vi "Run Bitfile.vi"() -> ()   [LabVIEW 2011]
uses:
  <vilib>/Platform/TimedLoop/XDataNode/timing_clust.ctl
  <vilib>/Platform/TimedLoop/XDataNode/nitl_modes.ctl
  <vilib>/Platform/TimedLoop/XDataNode/wakeup.ctl
  <vilib>/FPGAPlugInAG/sbRIO-9606/niLvFpga_Open_sbRIO-9606.vi
  <vilib>/rvi/interface/common/dynamic/niFpgaDynamicAddResources.vi
  <vilib>/Utility/error.llb/Error Cluster From Error Code.vi
  <vilib>/rvi/errors/niLvFpgaAdjustHostInterfaceError.vi
  <vilib>/FPGAPlugInAG/Dynamic/niLvFpga_Close_Dynamic.vi
  <vilib>/Platform/TimedLoop/XDataNode/XDataNode.xnode
  <vilib>/rvi/interface/nirviOpenFPGA/nirviOpenFPGA.xnode
  FPGA Bitfiles/natcar_FPGATarget_Top-Level_610FB000.lvbitx
  <vilib>/rvi/interface/nirviReadWriteControl/nirviReadWriteControl.xnode
  <vilib>/rvi/interface/nirviCloseFPGA/nirviCloseFPGA.xnode
  <vilib>/Platform/TimedLoop/XDataNode/XDNodeRunTimeDep.lvlib
  NiFpgaLv.dll
  <vilib>/rvi/interface/Simulation/niFpgaSimulationCallBeginRW.vi
panel:
  out "straight":bool
  in  "slow":u16=45 max=100 step=1
  in  "fast":u16=53 max=100 step=1
  out "using SL,SR":bool
  out "Error from SL,SR":dbl(graph)
  out "from SL,SR":dbl
  out "S5":bool
  out "S4":bool
  out "S2":bool
  out "S1":bool
  out "Raw Sensor Data":T1(graph)
  out "Go Duty":u16
  out "Servo 1e-7s":u32
  out "Line Error Graph":dbl(graph)
  out "Error (cm)":dbl
  in  "Steering Kp":dbl=270.0 min=0.0 max=1000.0 step=1.0
  out "really lost":bool
  out "line found":bool
  out "SC":bool
  out "S3":bool
  out "AI7":u16
  out "AI6":u16
  out "AI5":u16
  out "AI4":u16
  out "AI3":u16
  out "AI2":u16
  out "AI1":u16
  out "AI0":u16
  out "Speed Error":dbl(graph)
  in  "Offset":dbl=35.0 min=0.0 max=30.0 step=0.1
  out "Velocity counts":u32
  out "V [m/s]":dbl
  in  "RUN!":bool
  in  "Stop":bool
  in  "Kff":dbl=6.0 min=0.0 max=10.0 step=0.1
  in  "uBlaze Reset":bool
  in  "Steering ON 1e-7s":u32=15000 min=10240 max=19650 step=100
  in  "Steering":bool
  in  "Throttle":bool
  in  "GO frequency (Hz)":u16=1000 min=10 max=10000 step=10
  in  "GO duty":u16 max=100 step=1
  in  "Vdes [m/s]":dbl min=0.0 max=5.0 step=0.1
  in  "Speed Ki":dbl=0.1 min=0.0 max=2.0 step=0.01
  in  "Throttle ON":bool
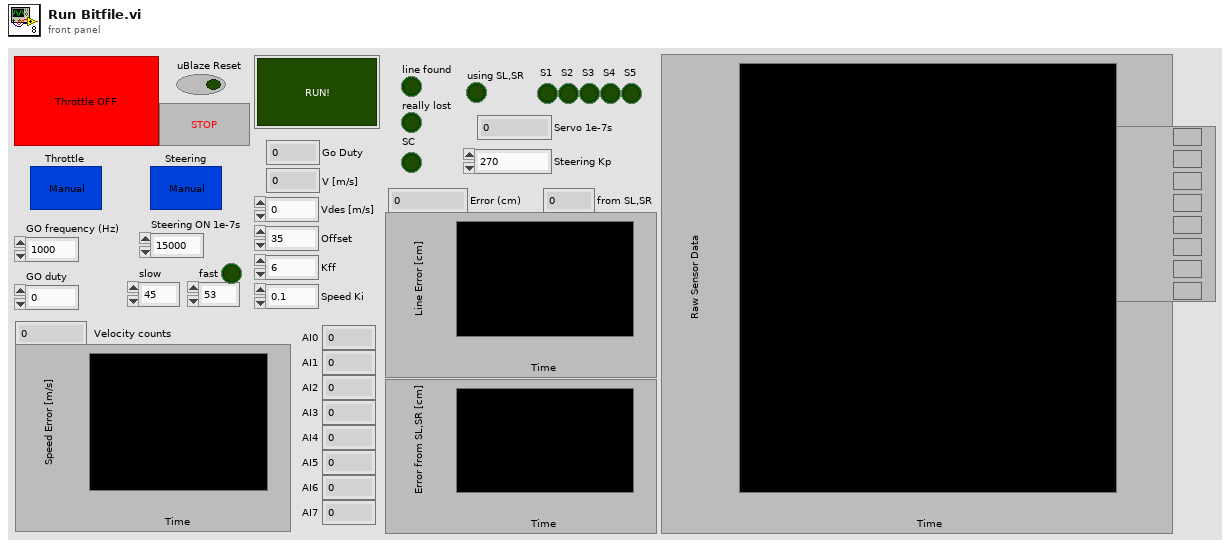
[diagram p1: front panel]
types:
  T1 = cluster{"AI0":u16, "AI1":u16, "AI2":u16, "AI3":u16, "AI4":u16, "AI5":u16, "AI6":u16, "AI7":u16}
  T2 = typedef "XDNodeRunTimeDep.lvlib/timing_clust.ctl" = cluster{"Expected End [f-1]":u64, "Actual End [f-1]":u64, "Finished Late? [f-1]":bool, "Expected End [i-1]":u64, "Actual End [i-1]":u64, "Finished Late? [i-1]":bool, "Expected Start [i]":u64, "Actual Start [i]":u64, "Expected Start [f]":u64, "Actual Start [f]":u64, "Source Name":string, "Structure Name":string, "Period":i64, "Deadline":i64, "Offset":i64, "Start":i64, "Priority":i32, "Timeout":i32, "Mode":T3, "Wakeup Reason":T4, "Error":errorcluster, "Source Type":string, "Secondary Source Type":string, "Global End Time":u64, "Global Start Time":u64, "Frame Duration":u64, "Iteration Duration":u64, "Assigned CPU":i32, "I/O Scan Engine Mode":u32}
  T3 = typedef "XDNodeRunTimeDep.lvlib/nitl_modes.ctl" = enum32{"No Change", "Process missed periods, maintain original phase", "Discard missed periods, maintain original phase", "Process missed periods, ignore original phase", "Discard missed periods, ignore original phase"}
  T4 = typedef "XDNodeRunTimeDep.lvlib/wakeup.ctl" = enum32{"Normal", "Aborted", "Asynchronous wakeup", "Timing source error", "Timed loop error", "Timeout"}
  T5 = cluster{"AI5":u16, "AI6":u16, "AI7":u16, "AI2":u16, "AI1":u16, "AI3":u16, "AI4":u16, "AI0":u16}
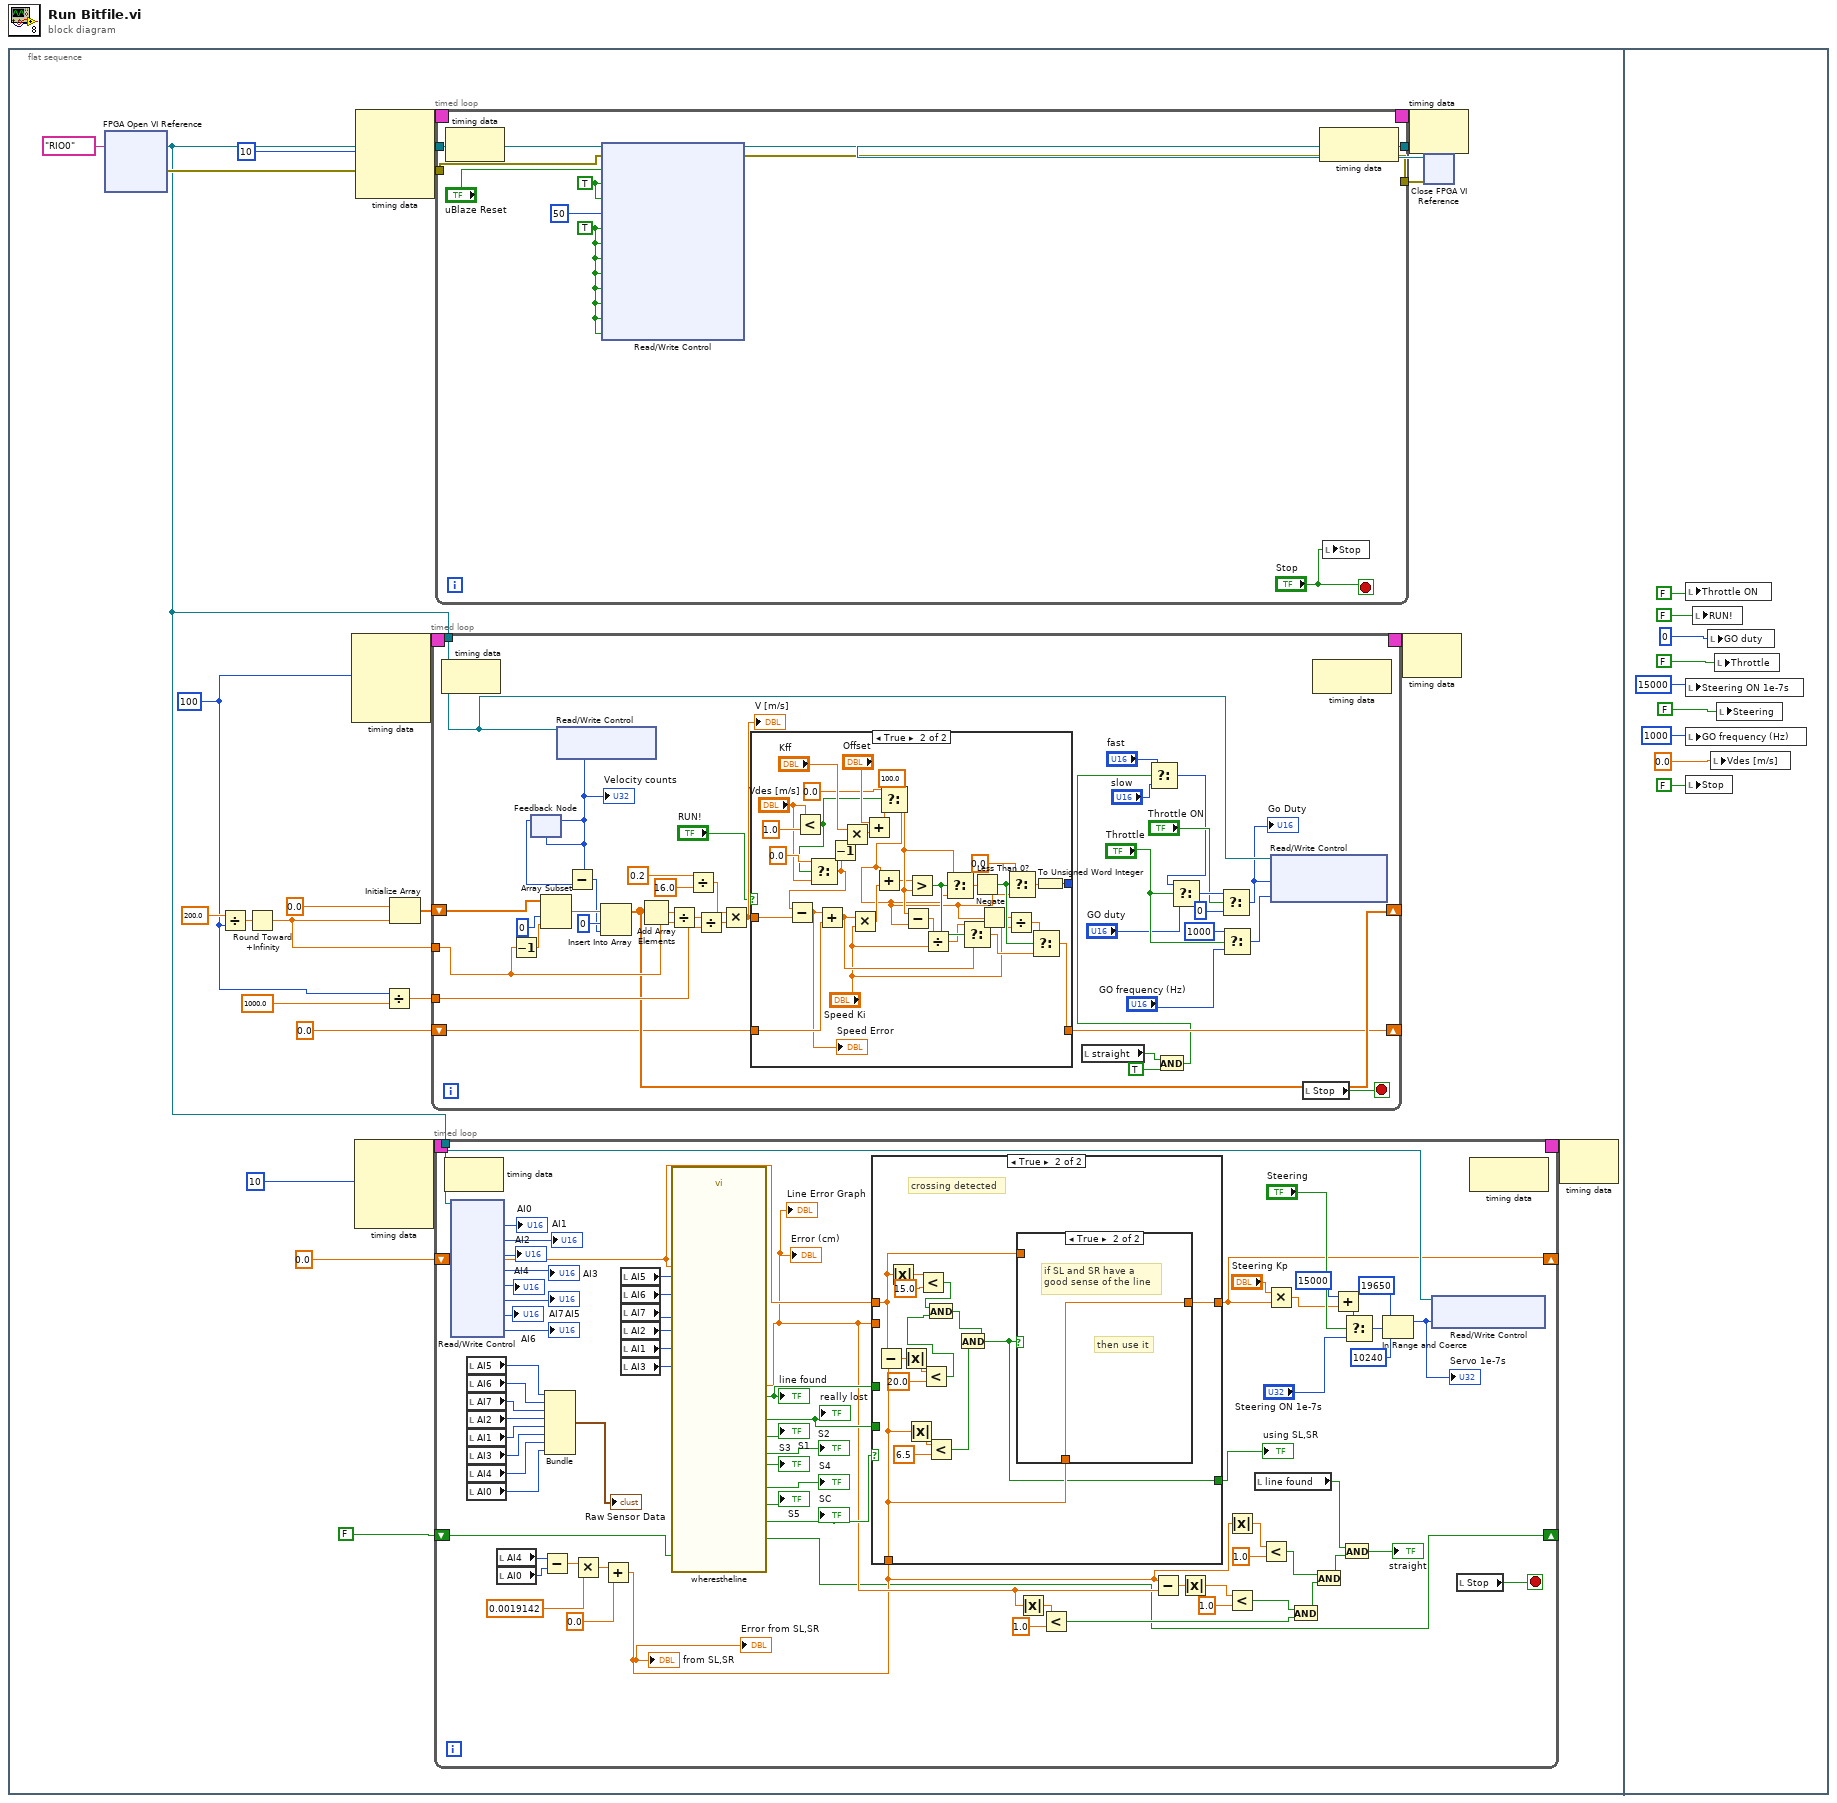
[diagram p0: block diagram]
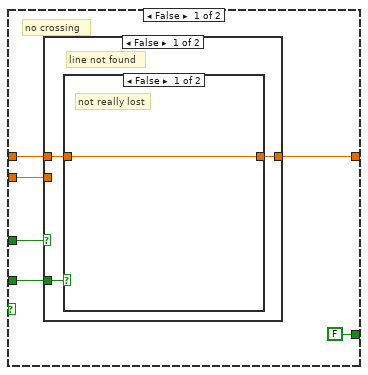
[diagram p2: hidden frame]
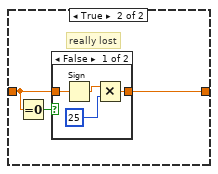
[diagram p3: hidden frame]
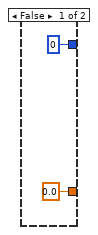
[diagram p7: hidden frame]
diagram:
  n1 = flat-sequence {
    frame #0 {
      w4 = i64 100 ("Period")
      n2 = xnode "FPGA Open VI Reference"("resource name"=tag "RIO0") -> ("FPGA VI Reference Out"=w3:refnum<k20>, "error out"=w17:errorcluster)  [unwired: 1 in]
      n3 = Divide(x=200.0, y=w4) -> (x/y=w11:dbl)
      n4 = Round Toward +Infinity(x=w11) -> (ceil(x): smallest int >= x=w10:dbl)
      n5 = node-c288(w4) -> (w24:T2)  [unwired: 3 in]
      n6 = node-c288(i64 10 ("Period")) -> (w22:T2)  [unwired: 3 in]
      n7 = node-c288(i64 10 ("Period")) -> (w20:T2)  [unwired: 3 in]
      n8 = Divide(x=w4, y=1000.0) -> (x/y=w6:dbl)
      n9 = Initialize Array(0.0 ("element"), w10) -> (w14:dbl[])
      n10 = timed-loop {
        timing: w24 -> [_]
        timing-out: [_] -> w23
        shift-right: [w187] -> _
        shift-left: w14 -> [w186]
        tunnel: w10 -> [w189]
        tunnel: w6 -> [w188]
        shift-right: [w184] -> _
        shift-left: 0.0 -> [w185]
        tunnel: w3 -> [w183]
        stop <- w182 stop-if-true
        n11 = node-c288() -> ()  [unwired: 1 in, 1 out]
        n12 = Decrement(x=w189) -> (x-1=w171:dbl)
        n13 = Array Subset(array=w186, index=0, length=w171) -> (w163:dbl[])
        n14 = xnode "Read/Write Control"("FPGA VI Reference In"=w183) -> ("Velocity counts"=w159:u32)  [unwired: 1 in, 2 out]
        "Velocity counts" <- w159
        n15 = feedback #1(w159) -> (w160:u32)
        n16 = feedback-in #1(w159) -> ()
        n17 = Subtract(x=w159, y=w160) -> (x-y=w162:u32)
        n18 = Insert Into Array(array=w163, index=0, new element=w162) -> (w187:dbl[])
        n19 = Add Array Elements(numeric array=w187) -> (sum=w161:dbl)
        n20 = Divide(x=w161, y=w189) -> (x/y=w169:dbl)
        n21 = Divide(x=0.2, y=16.0) -> (x/y=w165:dbl)
        n22 = Divide(x=w169, y=w188) -> (x/y=w166:dbl)
        n23 = Multiply(x=w165, y=w166) -> (x*y=w164:dbl)
        "V [m/s]" <- w164
        n24 = case shown="True" "RUN!" {
          tunnel: w185 -> [_ w223]
          tunnel: [0.0 w222] -> w184
          tunnel: [u16 0 w221] -> _
          tunnel: w164 -> [_ w220]
          frame False {
          }
          frame True {
            w214 = 100.0 ("y")
            n25 = Less?(x="Vdes [m/s]", y=1.0) -> (x < y?=w196:bool)
            n26 = Select(t=0.0, s=w196, f="Vdes [m/s]") -> (s? t:f=w197:dbl)
            n27 = Subtract(x=w197, y=w220) -> (x-y=w192:dbl)
            "Speed Error" <- w192
            n28 = Add(x=w192, y=w223) -> (x+y=w207:dbl)
            n29 = Decrement(x=w197) -> (x-1=w198:dbl)
            n30 = Multiply(x="Kff", y=w198) -> (x*y=w201:dbl)
            n31 = Multiply(x=w207, y="Speed Ki") -> (x*y=w219:dbl)
            n32 = Add(x="Offset", y=w201) -> (x+y=w194:dbl)
            n33 = Select(t=0.0, s=w196, f=w194) -> (s? t:f=w193:dbl)
            n34 = Add(x=w193, y=w219) -> (x+y=w210:dbl)
            n35 = Subtract(x=w214, y=w193) -> (x-y=w213:dbl)
            n36 = Greater?(x=w210, y=w214) -> (0:w215:bool)
            n37 = Divide(x=w213, y="Speed Ki") -> (x/y=w212:dbl)
            n38 = Select(t=w214, s=w215, f=w193) -> (s? t:f=w216:dbl)
            n39 = Select(t=w212, s=w215, f=w207) -> (s? t:f=w205:dbl)
            n40 = Less Than 0?(x=w216) -> (x < 0?=w211:bool)
            n41 = Negate(x=w193) -> (-x=w209:dbl)
            n42 = Divide(x=w209, y="Speed Ki") -> (x/y=w208:dbl)
            n43 = Select(t=0.0, s=w211, f=w193) -> (s? t:f=w206:dbl)
            n44 = Select(t=w208, s=w211, f=w205) -> (s? t:f=w222:dbl)
            n45 = To Unsigned Word Integer(number=w206) -> (unsigned 16bit integer=w221:u16)
          }
        }
        n46 = local read "straight"() -> (w154:bool)
        n47 = And(x=w154, y=TRUE) -> (x .and. y?=w153:bool)
        n48 = Select(t="fast", s=w153, f="slow") -> (s? t:f=w155:u16)
        n49 = Select(t=w155, s="Throttle", f="GO duty") -> (s? t:f=w175:u16)
        n50 = Select(t=w175, s="Throttle ON", f=u16 0 ("t")) -> (s? t:f=w174:u16)
        "Go Duty" <- w174
        n51 = Select(t=u16 1000, s="Throttle", f="GO frequency (Hz)") -> (s? t:f=w177:u16)
        n52 = xnode "Read/Write Control"("FPGA VI Reference In"=w183, "GO duty (100*%)"=w174, "GO frequency (Hz)"=w177) -> ()  [unwired: 1 in, 2 out]
        n53 = local read "Stop"() -> (w182:bool)
        n54 = node-c288() -> ()  [unwired: 1 in, 1 out]
      }
      n55 = timed-loop {
        timing: w22 -> [_]
        timing-out: [_] -> w21
        tunnel: w3 -> [w84]
        shift-right: [w83] -> _
        shift-left: 0.0 -> [w95]
        shift-right: [w41] -> _
        shift-left: FALSE -> [w42]
        stop <- w108 stop-if-true
        n56 = node-c288() -> ()  [unwired: 1 in, 1 out]
        n57 = xnode "Read/Write Control"("FPGA VI Reference In"=w84) -> ("AI0"=→"AI0":u16, "AI1"=→"AI1":u16, "AI2"=→"AI2":u16, "AI3"=→"AI3":u16, "AI4"=→"AI4":u16, "AI5"=→"AI5":u16, "AI6"=→"AI6":u16, "AI7"=→"AI7":u16)  [unwired: 1 in, 2 out]
        n58 = local read "AI5"() -> (w80:u16)
        n59 = local read "AI6"() -> (w79:u16)
        n60 = local read "AI7"() -> (w78:u16)
        n61 = local read "AI2"() -> (w77:u16)
        n62 = local read "AI1"() -> (w73:u16)
        n63 = local read "AI3"() -> (w74:u16)
        n64 = local read "AI4"() -> (w75:u16)
        n65 = local read "AI0"() -> (w76:u16)
        n66 = local read "AI4"() -> (w64:u16)
        n67 = local read "AI0"() -> (w63:u16)
        n68 = Subtract(x=w64, y=w63) -> (x-y=w62:dbl)
        n69 = Bundle("AI5"=w80, "AI6"=w79, "AI7"=w78, "AI2"=w77, "AI1"=w73, "AI3"=w74, "AI4"=w75, "AI0"=w76) -> (→"Raw Sensor Data":T5)  [unwired: 1 in]
        n70 = Multiply(x=w62, y=0.0019142) -> (x*y=w61:dbl)
        n71 = Add(x=w61, y=0.0) -> (x+y=w51:dbl)
        "from SL,SR" <- w51
        "Error from SL,SR" <- w51
        n72 = local read "AI5"() -> (w71:u16)
        n73 = local read "AI6"() -> (w70:u16)
        n74 = local read "AI7"() -> (w69:u16)
        n75 = local read "AI2"() -> (w68:u16)
        n76 = local read "AI1"() -> (w67:u16)
        n77 = local read "AI3"() -> (w66:u16)
        n78 = call "wherestheline.vi"("SCin"=w66, "S1in"=w71, "S2in"=w70, "S3in"=w69, "S4in"=w68, "S5in"=w67, "last error"=w95, "crossing started last time"=w42) -> ("crossing started"=w41:bool, "SC"=w92:bool, "error"=w54:dbl, "line found"=w96:bool, "really lost"=w93:bool, "S1"=→"S1":bool, "S2"=→"S2":bool, "S3"=→"S3":bool, "S4"=→"S4":bool, "S5"=→"S5":bool)  [unwired: 10 in]
        "SC" <- w92
        "line found" <- w96
        "really lost" <- w93
        "Error (cm)" <- w54
        "Line Error Graph" <- w54
        n79 = case shown="True" w92 {
          tunnel: w96 -> [w115 _]
          tunnel: w95 -> [w114 w130]
          tunnel: w54 -> [w113 _]
          tunnel: [w112 w131] -> w83
          tunnel: w93 -> [w111 _]
          tunnel: w51 -> [_ w132]
          tunnel: [FALSE w129] -> w40
          frame False {
            # "no crossing"
            n80 = case shown="False" w115 {
              tunnel: w114 -> [w117 _]
              tunnel: w113 -> [_ w128]
              tunnel: [w116 w128] -> w112
              tunnel: w111 -> [w118 _]
              frame False {
                # "line not found"
                n81 = case shown="False" w118 {
                  tunnel: [w119 w121] -> w116
                  tunnel: w117 -> [w119 w120]
                  frame False {
                    # "not really lost"
                  }
                  frame True {
                    # "really lost"
                    n82 = Equal To 0?(x=w120) -> (x = 0?=w122:bool)
                    n83 = case shown="False" w122 {
                      tunnel: [w123 w127] -> w121
                      tunnel: w120 -> [w126 w127]
                      frame False {
                        n84 = Sign(1:w126) -> (0:w125:dbl)
                        n85 = Multiply(x=w125, y=u16 25) -> (x*y=w123:dbl)
                      }
                      frame True {
                      }
                    }
                  }
                }
              }
              frame True {
                # "line is found"
              }
            }
          }
          frame True {
            # "crossing detected"
            n86 = Subtract(x=w130, y=w132) -> (x-y=w140:dbl)
            n87 = Absolute Value(x=w130) -> (abs(x)=w143:dbl)
            n88 = Absolute Value(x=w140) -> (abs(x)=w139:dbl)
            n89 = Absolute Value(x=w132) -> (abs(x)=w134:dbl)
            n90 = Less?(x=w143, y=15.0) -> (x < y?=w141:bool)
            n91 = Less?(x=w139, y=20.0) -> (x < y?=w137:bool)
            n92 = And(x=w141, y=w137) -> (x .and. y?=w136:bool)
            n93 = Less?(x=w134, y=6.5) -> (x < y?=w133:bool)
            n94 = And(x=w136, y=w133) -> (x .and. y?=w129:bool)
            n95 = case shown="True" w129 {
              tunnel: w132 -> [_ w145]
              tunnel: [w144 w145] -> w131
              tunnel: w130 -> [w144 _]
              frame False {
              }
              frame True {
                # "then use it"
                # "if SL and SR have a\ngood sense of the line"
              }
            }
          }
        }
        "using SL,SR" <- w40
        n96 = Absolute Value(x=w54) -> (abs(x)=w53:dbl)
        n97 = Less?(x=w53, y=1.0) -> (x < y?=w49:bool)
        n98 = Subtract(x=w51, y=w54) -> (x-y=w58:dbl)
        n99 = Absolute Value(x=w58) -> (abs(x)=w57:dbl)
        n100 = Absolute Value(x=w51) -> (abs(x)=w50:dbl)
        n101 = Less?(x=w57, y=1.0) -> (x < y?=w48:bool)
        n102 = local read "line found"() -> (w44:bool)
        n103 = Less?(x=w50, y=1.0) -> (x < y?=w46:bool)
        n104 = Multiply(x="Steering Kp", y=w83) -> (x*y=w65:dbl)
        n105 = And(x=w48, y=w49) -> (x .and. y?=w47:bool)
        n106 = And(x=w46, y=w47) -> (x .and. y?=w45:bool)
        n107 = Add(x=u32 15000, y=w65) -> (x+y=w90:u32)
        n108 = And(x=w44, y=w45) -> (x .and. y?=→"straight":bool)
        n109 = Select(t=w90, s="Steering", f="Steering ON 1e-7s") -> (s? t:f=w88:u32)
        n110 = In Range and Coerce(upper limit=u32 19650, x=w88, lower limit=u32 10240) -> (coerced(x)=w85:u32)  [unwired: 1 out]
        "Servo 1e-7s" <- w85
        n111 = xnode "Read/Write Control"("FPGA VI Reference In"=w84, "Steering ON 1e-7s"=w85) -> ()  [unwired: 1 in, 2 out]
        n112 = local read "Stop"() -> (w108:bool)
        n113 = node-c288() -> ()  [unwired: 1 in, 1 out]
      }
      n114 = timed-loop {
        tunnel: w3 -> [w33]
        tunnel: [w32] -> w18
        tunnel: w17 -> [w30]
        tunnel: [w29] -> w16
        timing: w20 -> [_]
        timing-out: [_] -> w19
        stop <- "Stop" stop-if-true
        w25 = TRUE ("Enable AI0")
        w28 = TRUE ("manual steering")
        n115 = node-c288() -> ()  [unwired: 1 in, 1 out]
        n116 = xnode "Read/Write Control"("FPGA VI Reference In"=w33, "error in"=w30, "uBlaze Reset"="uBlaze Reset", "manual steering"=w28, "manual throttle"=w28, "Steering frequency (Hz)"=u16 50, "Enable AI0"=w25, "Enable AI1"=w25, "Enable AI2"=w25, "Enable AI3"=w25, "Enable AI4"=w25, "Enable AI5"=w25, "Enable AI6"=w25, "Enable AI7"=w25) -> ("FPGA VI Reference Out"=w32:refnum<k20>, "error out"=w29:errorcluster)
        n117 = node-c288() -> ()  [unwired: 1 in, 1 out]
        n118 = local write "Stop"("Stop") -> ()
      }
      n119 = node-c288(w23) -> ()  [unwired: 1 out]
      n120 = node-c288(w19) -> ()  [unwired: 1 out]
      n121 = xnode "Close FPGA VI Reference"("FPGA VI Reference In"=w18, "error in"=w16) -> ()  [unwired: 1 out]
      n122 = node-c288(w21) -> ()  [unwired: 1 out]
    }
    frame #1 {
      n123 = local write "Throttle ON"(FALSE ("Throttle ON")) -> ()
      n124 = local write "Steering ON 1e-7s"(u32 15000 ("Steering ON 1e-7s")) -> ()
      n125 = local write "GO frequency (Hz)"(u16 1000 ("GO frequency (Hz)")) -> ()
      n126 = local write "Stop"(FALSE ("Stop")) -> ()
      n127 = local write "RUN!"(FALSE ("START!")) -> ()
      n128 = local write "GO duty"(u16 0 ("GO duty (100*%)")) -> ()
      n129 = local write "Vdes [m/s]"(0.0 ("Desired Speed [m/s]")) -> ()
      n130 = local write "Throttle"(FALSE ("Automatic Throttle")) -> ()
      n131 = local write "Steering"(FALSE ("Automatic Steering")) -> ()
    }
  }
